vi "Global - Data UDP.vi"() -> ()   [LabVIEW 2019]
uses:
  UDP - Status.ctl
  UDP - Event.ctl
panel:
  in  "Loop 16":bool
  in  "Loop 15":bool
  in  "Loop 14":bool
  in  "Loop 13":bool
  in  "Loop 12":bool
  in  "Loop 11":bool
  in  "Loop 10":bool
  in  "Loop 9":bool
  in  "Loop 8":bool
  in  "Loop 7":bool
  in  "Loop 6":bool
  in  "Loop 5":bool
  in  "Loop 4":bool
  in  "Loop 3":bool
  in  "Loop 2":bool
  in  "Loop 1":bool
  in  "V1":bool
  in  "DL Sens":T1
  in  "Local IP":string
  in  "Controller":T2
  in  "DL":T2
  in  "Channels":T2
  out "System":T3
  in  "Event":T4 items=["Stop", "Running", "PID", "Up Limit", "Down Limit", "Load Limit"]
  in  "Status":T5 items=["Stop", "Ramp Up", "Ramp Down", "Jog Up", "Jog Down", "PID Mode", "PID Ramp"]
  in  "PID":T6={"SP"=-2.7823365e-08, "PV"=-3.023652e-13, "kP"=8.5432666e-24, "kI"=2.29252e-41, "kD"=1.570387e-38, "FF"=25.0, "Err Band"=0.0, "Max"=15, "Min"=-7, "Ts"=1886611780, "Out"=0, "Mode"=0}
  in  "ADC":T7={"Active Ch"=[255, 255, 255, 0, 0, 0, 0, 0], "Filter Type"=2, "Post Filter"=[1, 1, 1, 1, 0, 200, 66, 184], "Gain"=[0, 0, 0, 0, 0, 122, 68, 0], "FS"=32, "IntOC"=0, "IntFC"=255, "SysOC"=255, "Cofficient"=[1.0, 1.0, 1.0, 1.0, 1.0, 1.0, 1.0, 1.0], "K"=[1.2450000047683716, 1.2450000047683716], "Max"=1048576}
  in  "Sensor":T1
  in  "Test":T8
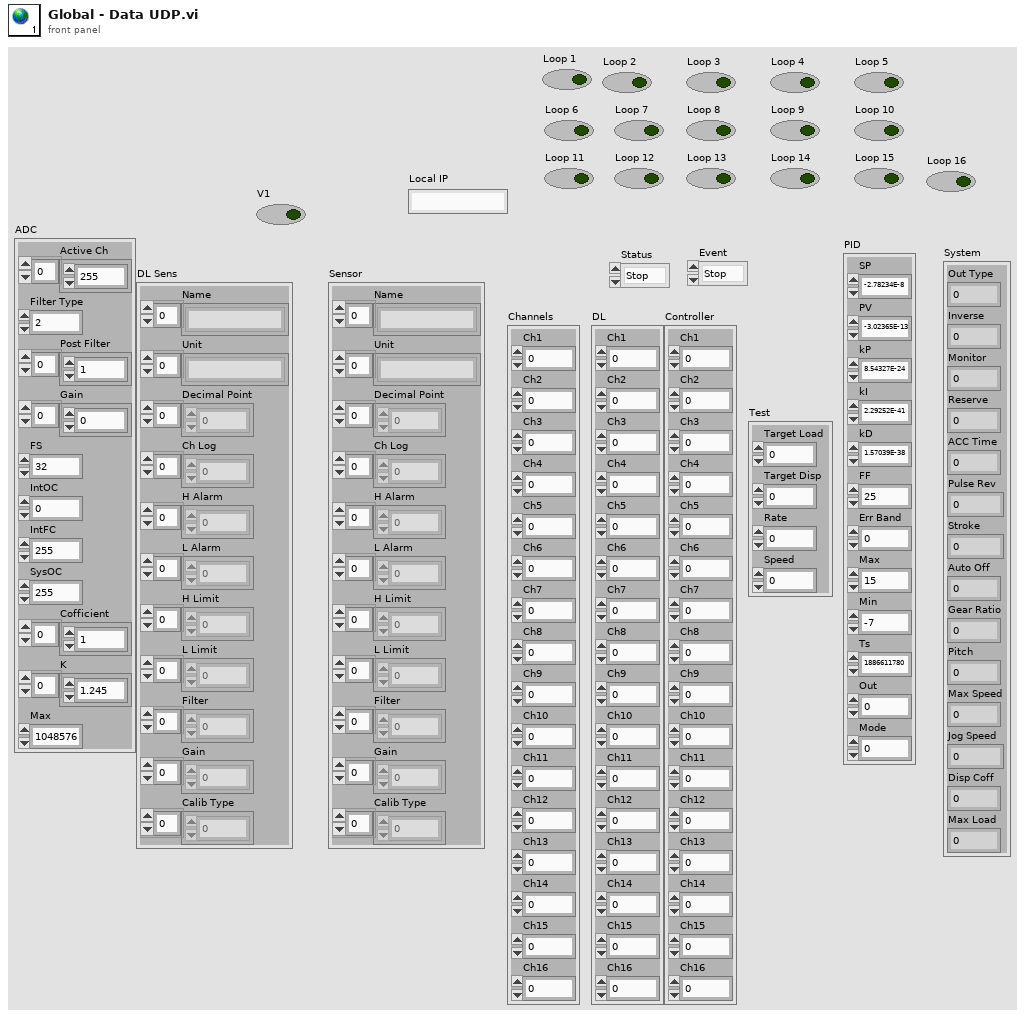
[diagram p1: front panel]
types:
  T1 = cluster{"Name":string[], "Unit":string[], "Decimal Point":u8[], "Ch Log":u8[], "H Alarm":u8[], "L Alarm":u8[], "H Limit":sgl[], "L Limit":sgl[], "Filter":u8[], "Gain":u8[], "Calib Type":u32[]}
  T2 = cluster{"Ch1":sgl, "Ch2":sgl, "Ch3":sgl, "Ch4":sgl, "Ch5":sgl, "Ch6":sgl, "Ch7":sgl, "Ch8":sgl, "Ch9":sgl, "Ch10":sgl, "Ch11":sgl, "Ch12":sgl, "Ch13":sgl, "Ch14":sgl, "Ch15":sgl, "Ch16":sgl}
  T3 = cluster{"Out Type":u8, "Inverse":u8, "Monitor":u8, "Reserve":u8, "ACC Time":u32, "Pulse Rev":u32, "Stroke":u32, "Auto Off":u32, "Gear Ratio":sgl, "Pitch":sgl, "Max Speed":u32, "Jog Speed":u32, "Disp Coff":sgl, "Max Load":u32}
  T4 = typedef "UDP - Event.ctl" = u16
  T5 = typedef "UDP - Status.ctl" = u16
  T6 = cluster{"SP":sgl, "PV":sgl, "kP":sgl, "kI":sgl, "kD":sgl, "FF":sgl, "Err Band":sgl, "Max":i32, "Min":i32, "Ts":u32, "Out":i32, "Mode":u8}
  T7 = cluster{"Active Ch":u8[], "Filter Type":u8, "Post Filter":u8[], "Gain":u8[], "FS":u16, "IntOC":u8, "IntFC":u8, "SysOC":u8, "Cofficient":dbl[], "K":dbl[], "Max":i32}
  T8 = cluster{"Target Load":sgl, "Target Disp":sgl, "Rate":sgl, "Speed":sgl}
diagram:
